vi "WriteFile.vi"   [LabVIEW 2021]
uses:
  Classes/WOFile/WOFile.lvclass
  Classes/RWFile/RWFile.lvclass
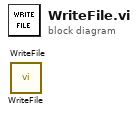
[diagram p0: block diagram]
diagram:
  n1 = call "WriteFile.vi"() -> ()  [unwired: 10 in, 2 out]
  n2 = call "WriteFile.vi"() -> ()  [unwired: 10 in, 2 out]
